vi "To Array.vi"() -> ()   [LabVIEW 2015, in "Point.lvclass"]
uses:
  Point.lvclass
  Point.lvclass/Point.ctl
panel:
  out "Point":dbl[](array[numeric])
  out "error out":errorcluster
  in  "error in (no error)":errorcluster
  in  "Point.lvclass":refnum<class "Point.lvclass">
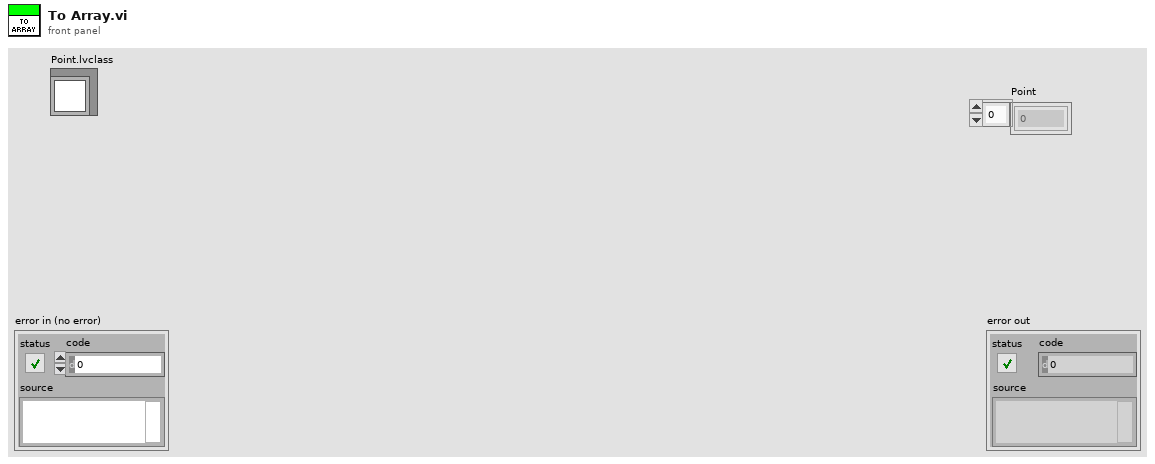
[diagram p1: front panel]
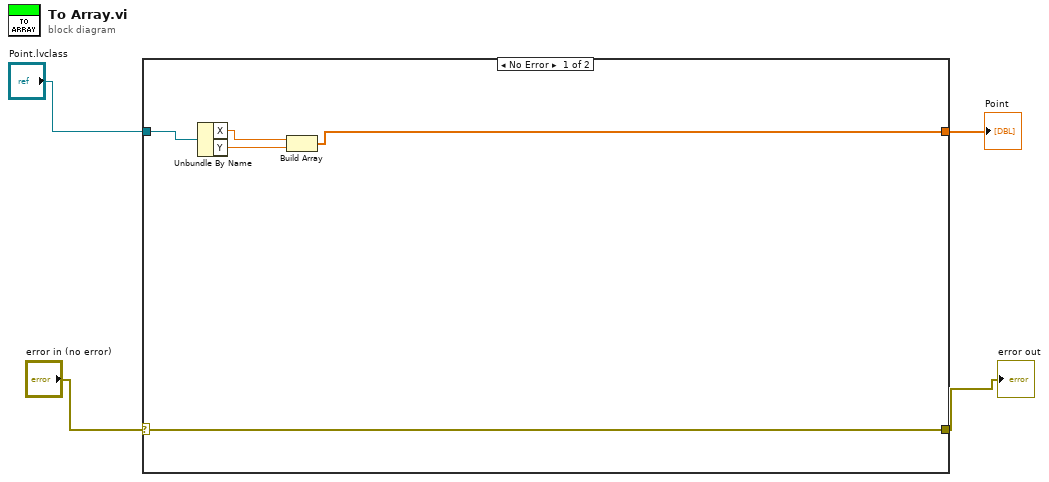
[diagram p0: block diagram]
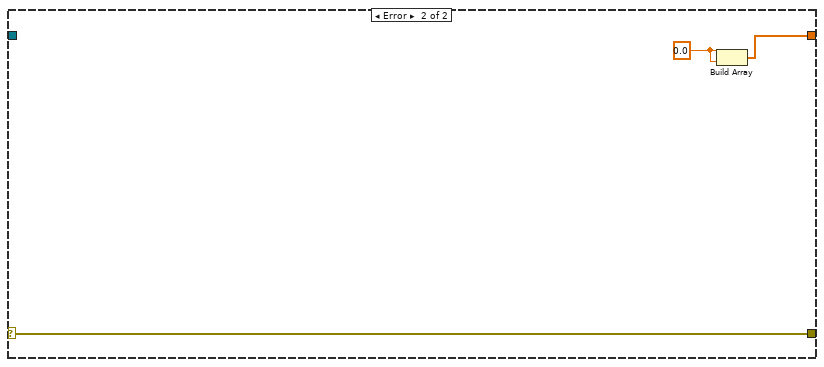
[diagram p2: hidden frame]
diagram:
  n1 = case shown="No Error" "error in (no error)" {
    selector: "error in (no error)" -> [w9 w12]
    tunnel: [w9 w12] -> w3
    tunnel: [w5 w10] -> w2
    tunnel: "Point.lvclass" -> [w8 _]
    frame No Error {
      n2 = Unbundle By Name(w8) -> ("X"=w7:dbl, "Y"=w6:dbl)
      n3 = Build Array(w7, w6) -> (w5:dbl[])
    }
    frame Error {
      w11 = 0.0
      n4 = Build Array(w11, w11) -> (w10:dbl[])
    }
  }
  "error out" <- w3
  "Point" <- w2
